vi "LoadControlPanel.vi"(8 "error in (no error)":errorcluster, 10 "Actor In":refnum<class "Actor.lvclass">, 11 "Stage_MadCityLabMicro in":refnum<class "Stage_MadCityLabMicro.lvclass">) -> (0 "error out":errorcluster, 3 "Stage_MadCityLabMicro out":refnum<class "Stage_MadCityLabMicro.lvclass">)   [LabVIEW 2020, in "Stage_MadCityLabMicro.lvlib" / "Stage_MadCityLabMicro.lvclass"]
uses:
  Stage_MadCityLabMicro.lvclass
  ViewController/StepMotorController/StepMotorController.lvclass
  <vilib>/ActorFramework/Actor/Actor.lvclass
  C:/Program Files/National Instruments/LabVIEW 2020/vi.lib/ActorFramework/Actor/Actor.lvclass
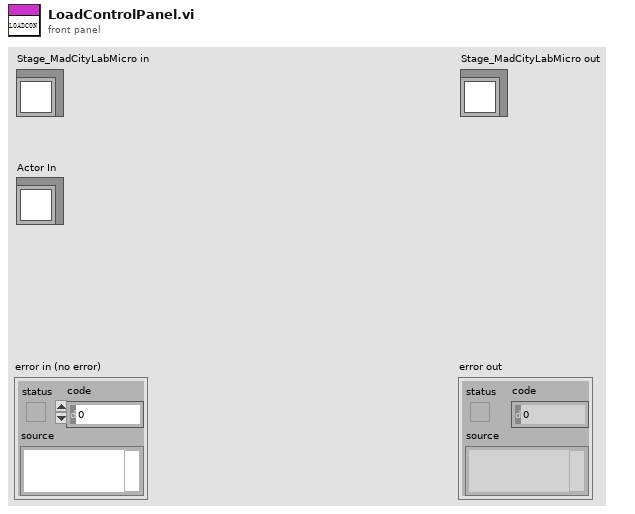
[diagram p1: front panel]
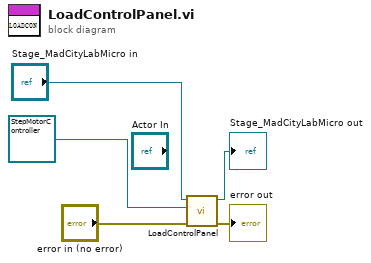
[diagram p0: block diagram]
diagram:
  n1 = call-parent "LoadControlPanel.vi"("error in (no error)"="error in (no error)", "Actor In"=refnum<class "StepMotorController.lvclass"> refnum ("StepMotorController.lvlib:StepMotorController.lvclass"), "GRMActor in"="Stage_MadCityLabMicro in") -> ("error out"=→"error out":errorcluster, "GRMActor out"=→"Stage_MadCityLabMicro out":refnum<class "Stage_MadCityLabMicro.lvclass">)  [unwired: 7 in]
